vi "Read Color.vi"(8 "error in (no error)":errorcluster, 11 "Color in":refnum<class "Color.lvclass">) -> (0 "error out":errorcluster, 2 "Color":refnum<k24>, 3 "Color out":refnum<class "Color.lvclass">)   [LabVIEW 2016, in "DataGrid.lvlib" / "Color.lvclass"]
doc: "Reads the .net color class for use with cells, columns, rows and other properties anywhere in .NET that uses color."
uses:
  <userlib>/LabVIEWdotNetDataGrid/source/Color/Color.lvclass
  System.Drawing
  <userlib>/LabVIEWdotNetDataGrid/source/Color/Color.lvclass/Color.ctl
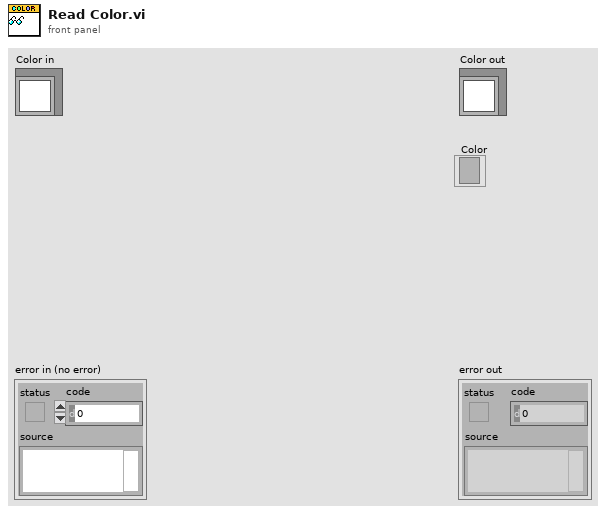
[diagram p1: front panel]
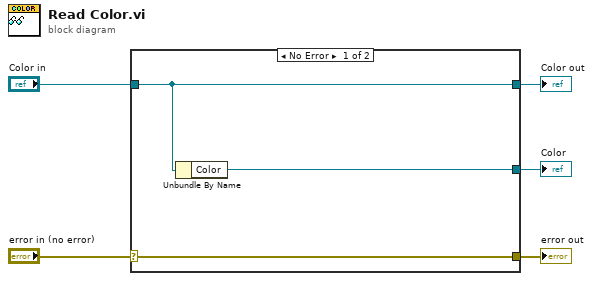
[diagram p0: block diagram]
diagram:
  n1 = case shown="No Error" "error in (no error)" {
    selector: "error in (no error)" -> [w8 w9]
    tunnel: [w8 w9] -> w4
    tunnel: [w7 w10] -> w2
    tunnel: "Color in" -> [w7 w10]
    tunnel: [w6 _] -> w1
    frame No Error {
      n2 = Unbundle By Name(w7) -> ("Color"=w6:refnum<k24>)
    }
    frame Error {
    }
  }
  "error out" <- w4
  "Color out" <- w2
  "Color" <- w1
